vi "XLP80_Datalog_CheckFileSize.vi"(8 "error in":errorcluster caption="error out", 11 "Filename":path) -> (0 "error OUT":errorcluster caption="error out")   [LabVIEW 2021]
doc: "Es wird der Dateiname überprüft und die erste Zeile des Files erzeugt (Spaltenbezeichnung). In der ersten Zeile stehen die Kanalnamen und die Zeit, in der zweiten Zeile stehen die Einheiten."
uses:
  XLP80_State_V001.llb/XLP80_State_TDefEnumStateDatalog.ctl
  XLP80_State_V001.llb/XLP80_State_Globals.vi
  XLP80_Globals/Globals_Settings_XLP80.vi
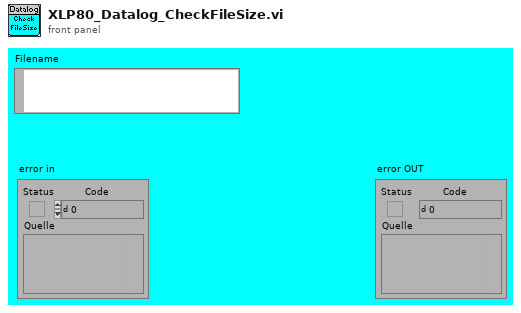
[diagram p1: front panel]
types:
  T1 = typedef "XLP80_State_TDefEnumStateDatalog.ctl" = enum16{"default", "StartLog", "Log", "StopLog", "NewFile"}
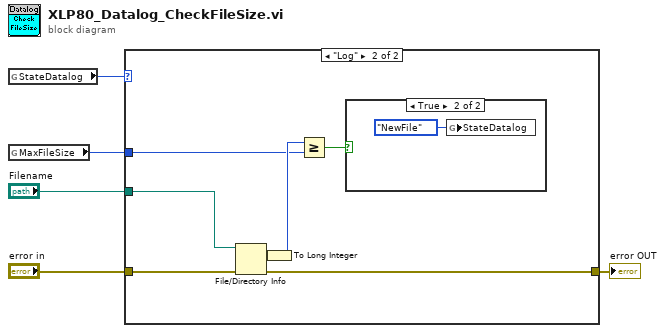
[diagram p0: block diagram]
diagram:
  n1 = global read "XLP80_State_Globals.vi" "StateDatalog"() -> (w2:T1)
  n2 = global read "Globals_Settings_XLP80.vi" "MaxFileSize"() -> (w1:i32)
  n3 = case shown="\"Log\"" w2 {
    tunnel: "error in" -> [w6 w13]
    tunnel: [w6 w12] -> w5
    tunnel: "Filename" -> [_ w11]
    tunnel: w1 -> [_ w9]
    frame Default {
    }
    frame "Log" {
      n4 = File/Directory Info(path=w11, error in=w13) -> (size=w7:i64, error out=w12:errorcluster)  [unwired: 5 out]
      n5 = To Long Integer(number=w7) -> (32bit integer=w10:i32)
      n6 = Greater Or Equal?(x=w10, y=w9) -> (x >= y?=w8:bool)
      n7 = case shown="True" w8 {
        frame False {
        }
        frame True {
          n8 = global write "XLP80_State_Globals.vi" "StateDatalog"(XLP80_State_TDefEnumStateDatalog."NewFile" ("StateDatalog")) -> ()
        }
      }
    }
  }
  "error OUT" <- w5
